vi "ParseAllVarsFile.vi"(0 "Path":path) -> (1 "CA output vars":T1, 2 "CA input vars":T2)   [LabVIEW 2010]
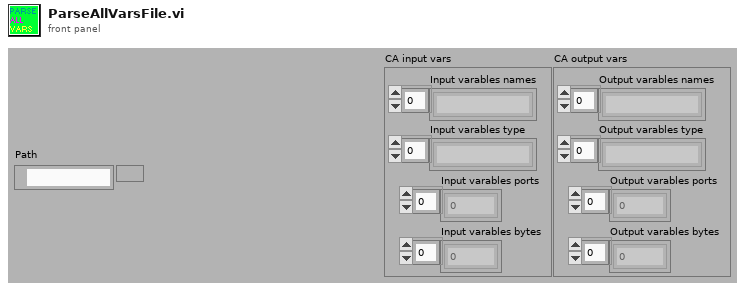
[diagram p1: front panel]
types:
  T1 = cluster{"Output varables names":string[], "Output varables type":string[], "Output varables ports":i32[], "Output varables bytes":i32[]}
  T2 = cluster{"Input varables names":string[], "Input varables type":string[], "Input varables ports":i32[], "Input varables bytes":i32[]}
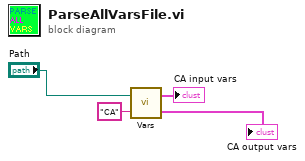
[diagram p0: block diagram]
diagram:
  n1 = call "Vars.vi"("name or relative path"="CA", "Path"="Path") -> ("output"=→"CA output vars":T1, "input"=→"CA input vars":T2)
